vi "Set_Reset_RW_LDAC.vi"(1 "error in":errorcluster, 2 "LDAC":bool, 3 "RW":bool) -> (0 "error out":errorcluster)   [LabVIEW 2017]
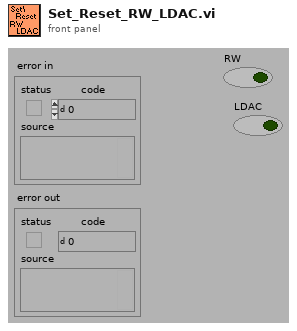
[diagram p1: front panel]
types:
  T1 = enum16{"Reset", "Update U1", "Update U2", "Update U3", "Read all"}
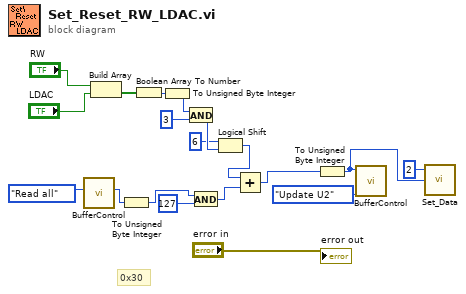
[diagram p0: block diagram]
diagram:
  # "0x30"
  n1 = call "BufferControl.vi"("Enum"=T1."Read all") -> ("U2BuffRead"=w9:u8)  [unwired: 3 in, 3 out]
  n2 = Build Array("RW", "LDAC") -> (w6:bool[])
  n3 = To Unsigned Byte Integer(number=w9) -> (unsigned 8bit integer=w12:u8)
  n4 = Boolean Array To Number(Boolean array=w6) -> (number=w5:u32)
  n5 = To Unsigned Byte Integer(number=w5) -> (unsigned 8bit integer=w4:u8)
  n6 = And(x=w4, y=u16 3) -> (x .and. y?=w3:u16)
  n7 = And(x=w12, y=u16 127) -> (x .and. y?=w11:u16)
  n8 = Logical Shift(y=u16 6, x=w3) -> (x << y=w2:u16)
  n9 = Add(x=w2, y=w11) -> (x+y=w10:u16)
  n10 = To Unsigned Byte Integer(number=w10) -> (unsigned 8bit integer=w16:u8)
  n11 = call "BufferControl.vi"("Enum"=T1."Update U2", "Data"=w16) -> ()  [unwired: 2 in, 4 out]
  n12 = call "Set_Data.vi"("Data"=w16, "Ch"=u8 2) -> ()  [unwired: 2 in, 1 out]
  "error out" <- "error in"
